vi "Dashboard Main.vi"() -> ()   [LabVIEW 2019]
uses:
  <vilib>/Utility/miscctls.llb/LVRowAndColumnTypeDef.ctl
  <vilib>/event_ctls.llb/eventvkey.ctl
  <vilib>/Rock Robotics/Network Tables/NT Read Numeric Array.vi
  <vilib>/Rock Robotics/WPI/Dashboard/WPI_DashboardLogging Global.vi
  <vilib>/Rock Robotics/Network Tables/NT Read Boolean.vi
  <vilib>/Rock Robotics/Network Tables/NT Write Boolean.vi
panel:
  in  "Camera Settings Right":T1={"Frame Rate"=30, "Compression"=30, "Size"=1, "DB Camera Config"=FALSE} {"Frame Rate" scale=1.0..30.0; "Compression" scale=100.0..-1.0; "Size" items=["640x480", "320x240", "160x120"]}
  in  "Camera Name Right":string(combo)="No Camera Selection"
  out "Camera Perf":string
  in  "Camera Settings":T1={"Frame Rate"=30, "Compression"=30, "Size"=1, "DB Camera Config"=FALSE} {"Frame Rate" scale=1.0..30.0; "Compression" scale=100.0..-1.0; "Size" items=["640x480", "320x240", "160x120"]}
  in  "TCP":refnum<k5>
  in  "Rec Mode":enum32{"Stop", "Record", "Playback"}(radio)
  out "Robot IP":string
  out "Image Message":string="Timeout in Camera Communications"
  in  "Dashboard Tab":T2(tab)
  in  "Dual Operators?":bool=TRUE
  in  "FT to IN":bool
  out "Target Acquired":bool
  out "Vision Enabled":bool
  out "NT Connection":bool
  out "MotorChart R":cluster{"Numeric":dbl, "Numeric":dbl}(graph)
  out "MotorChart L":cluster{"Numeric":dbl, "Numeric":dbl}(graph)
  out "MotorSliders R":cluster{"MotorSlide1":dbl, "MotorSlide2":dbl} {"MotorSlide2" scale=-1.0..1.0 scale format="%#_2e"; "MotorSlide1" scale=-1.0..1.0 scale format="%#_2e"}
  out "MotorSliders L":cluster{"MotorSlide1":dbl, "MotorSlide2":dbl} {"MotorSlide2" scale=-1.0..1.0 scale format="%#_2e"; "MotorSlide1" scale=-1.0..1.0 scale format="%#_2e"}
  out "JS1 Z":dbl(slide) scale=-1.0..1.0 scale format="%#_2e"
  out "JS1 Graph":cluster{"X":dbl, "Y":dbl}[](graph)
  out "JS1 Buttons":T3
  out "JS2 Z":dbl(slide) scale=-1.0..1.0 scale format="%#_2e"
  out "JS2 Graph":cluster{"X":dbl, "Y":dbl}[](graph)
  out "JS2 Buttons":T3
  out "Mode":T4(ring)=enum."Auto Disabled"
  out "Right Camera Perf":cluster{"Bandwidth (Mbps)":dbl, "FPS":dbl}
  in  "Select Auto":string(combo)="Select Autonomous ..."
  out "Target Distance":dbl
  out "Camera Image Right":T5(plugin-control)
  out "Skew":dbl caption="DB/String 1"
  out "Area":dbl caption="DB/String 1"
  out "Offset X":dbl
  out "Offset Y":dbl
  out "Bottom RPM":dbl caption="DB/String 1"
  out "Top RPM":dbl caption="DB/String 1"
  in  "Test Slider":dbl(slide) scale=0.0..100.0 scale format="%#_3g"
  in  "On/Off":bool caption="Solenoid"
  in  "Test Name":u16(ring) items=["Select the test to run..."]
  in  "Test Tree":string(tree)
  in  "Motor":cluster{"Value":dbl, "Enable":bool} {"Value" scale=-1.0..1.0 scale format="%#_3g"}
  out "Progress":T6 {"Test Progress" scale=0.0..100.0}
  in  "Rev/Fwd":cluster{"Forward":bool, "Reverse":bool}
  in  "Test Ring":u16(ring) items=["Monochrome", "Color"]
  out "Cmd Status":string
  in  "Execute Command":bool
  in  "Command Params":string[][](table)
  in  "Command Selection":i32(listbox)
  in  "CheckList":i32(listbox)
  out "Tree":string(tree)
  out "Camera Image":T5(plugin-control)
  out "Background":bool
  in  "Camera Name":string(combo)="No Camera Selection"
  # "HW"
  # "HW"
  # "Drive Motors"
  # "Front"
  # "Operator 1"
  # "Operator 2"
  # "Right"
  # "Left"
  # "Back"
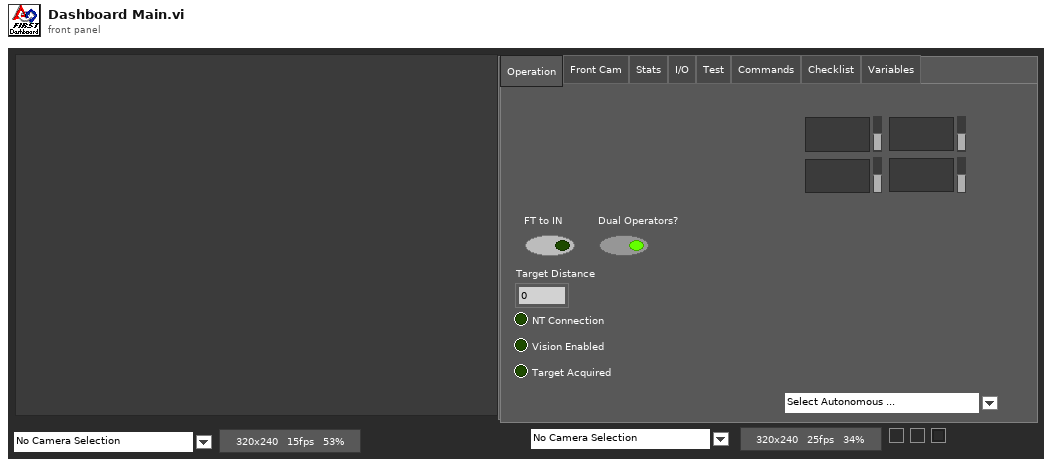
[diagram p1: front panel]
types:
  T1 = cluster{"Frame Rate":i32, "Compression":i32, "Size":u16, "DB Camera Config":bool}
  T2 = enum32{"Operation", "Front Cam", "Stats", "I/O", "Test", "Commands", "Checklist", "Variables"}
  T3 = cluster{bool, bool, bool, bool, bool, bool, bool, bool, bool, bool, bool, bool}
  T4 = enum8{"Tele-Op Disabled", "Tele-Op Enabled", "Auto Disabled", "Auto Enabled", "Test Disabled", "Test Enabled", "Disconnected", "No Code", "E-Stop"}
  T5 = typedef "IMAQ Image.ctl" = refnum<image>
  T6 = cluster{"Test Progress":u8, "Test Progress Text":string}
  T7 = cluster{"Save Path":path, "Interval (s)":dbl, "Keep":i32}
  T8 = enum32{"Drive", "Camera", "Basic", "Custom", "Test", "Commands", "Checklist", "Variables"}
  T9 = typedef "Image Type" = u32
  T10 = cluster{"IDs":cluster{"RPC field ID":u16, "Unique ID":u16}, "String":string}
  T11 = cluster{"Camera Image":refnum<vi>, "Dashboard Tab":refnum<vi>, "Background":refnum<vi>, "Rec Mode":refnum<vi>, "Test Slider":refnum<vi>, "On/Off ":refnum<vi>, "Test Ring":refnum<vi>, "Rev/Fwd":refnum<vi>, "Test Name":refnum<vi>, "Motor":refnum<vi>, "Progress":refnum<vi>, "CheckList":refnum<vi>, "Tree":refnum<vi>, "Test Tree":refnum<vi>, "Command Params":refnum<vi>, "Command Selection":refnum<vi>, "Execute Command":refnum<vi>, "Cmd Status":refnum<vi>, "Camera Settings":refnum<vi>, "Camera Name":refnum<vi>, "Camera Perf":refnum<vi>, "Camera Settings Right":refnum<vi>, "Camera Name Right":refnum<vi>, "Camera Image Right":refnum<vi>}
  T12 = cluster{"Global Rectangle":i32[], "Contours":cluster{"Contour Type":u32, "ROI Type":u32, "Points":i32[]}[]}
  T13 = cluster{"Camera Name Right":string, string, "Saved DB Images Info":cluster{"Save Path":path, "Interval (s)":dbl, "Keep":i32}}
  T14 = cluster{"Error Strings":string, "Disable Counts":cluster{u16, u16}, "Rail Faults":cluster{u16, u16, u16}, "Robot IP":string, "DB Mode":u8, "Event Info":cluster{"Name":string, "Type":u8, "Number":u16, "Replay":u8}}
  T15 = cluster{"Storage":cluster{"Disk Free":u64, "RAM Block":u32, "RAM free":u32}, "CPU Utilization":cluster{"CPU % ISR":sgl, "CPU % Time Crit":sgl, "CPU % Timed Str":sgl, "CPU % High":sgl, "CPU % Above":sgl, "CPU % Normal":sgl, "CPU % Low":sgl}, "CAN":cluster{"% Bus Utilization":sgl, "Bus Off Cnt":u32, "TX_FIFO Full Cnt":u32, "Receive Error Cnt":u8, "Transmit Error Cnt":u8}, "HID":cluster{"HID Outputs":u32, "Rumble Low":u16, "Rumble High":u16}[]}
  T16 = cluster{"Status bits":cluster{"Test Mode":bool, "Autonomous":bool, "Enabled":bool, "Code Start":bool, "Brownout":bool, "Reserved 2":bool, "Reserved 3":bool, "E-Stop":bool}, "Code Trace":cluster{"Disabled":bool, "TeleOp":bool, "Auto":bool, "Test":bool}, "Controller Type":enum16{"unknown", "cRIO", "roboRio"}, "Code?":enum16{"unknown", "noCode", "code"}, "Battery V":dbl}
  T17 = cluster{"Control Bits":cluster{"TestMode":bool, "Autonomous":bool, "Enabled":bool, "FMS Present":bool, bool, bool, bool, "E-Stop":bool}, "Team Station ":u8, "Countdown":sgl, "Joystick Values":cluster{"Axes":dbl[], "Buttons":bool[], "POVs":i16[]}[]}
  T18 = cluster{"Axes":dbl[], "Buttons":bool[], "POVs":i16[]}[]
  T19 = cluster{"Axes":dbl[], "Buttons":bool[], "POVs":i16[]}
  T20 = cluster{"Buttons[0]":bool, "Buttons[1]":bool, "Buttons[2]":bool, "Buttons[3]":bool, "Buttons[4]":bool, "Buttons[5]":bool, "Buttons[6]":bool, "Buttons[7]":bool, "Buttons[8]":bool, "Buttons[9]":bool, "Buttons[10]":bool, "Buttons[11]":bool}
  T21 = cluster{"Camera Name":string, string, "Saved DB Images Info":cluster{"Save Path":path, "Interval (s)":dbl, "Keep":i32}}
  T22 = cluster{"Operation":enum16{"Update", "Clear"}, "Color Box":u32}[]
  T23 = typedef "eventvkey.ctl" = enum16{"ASCII", "Enter", "Return", "Shift", "Ctrl", "Alt", "Cmd", "Opt", "Caps", "NumLock", "Clear", "Break", "Up", "Down", "Left", "Right", "Insert", "Delete", "Home", "End", "PageUp", "PageDown", "Escape", "Help", "Pause", "ScrollLock", "F1", "F2", "F3", "F4", "F5", "F6", "F7", "F8", "F9", "F10", "F11", "F12", "F13", "F14", "F15", "F16", "F17", "F18", "F19", "F20", "F21", "F22", "F23", "F24", "Play", "VolumeUp", "VolumeDown", "Mute", "Two Byte Char"}
  T24 = cluster{"Image Size":bool, "Image Type":bool, "Pixel Value":bool, "ROI Information":bool, "Zoom Factor":bool}
  T25 = cluster{"Operation":enum16{"Update", "Clear"}, "Color Box":u32}
  T26 = typedef "LVRowAndColumnTypeDef.ctl" = cluster{"Row":i32, "Column":i32}
  T27 = cluster{"Shift":bool, "Ctrl":bool, "Alt":bool, "Cmd":bool, "Opt":bool}
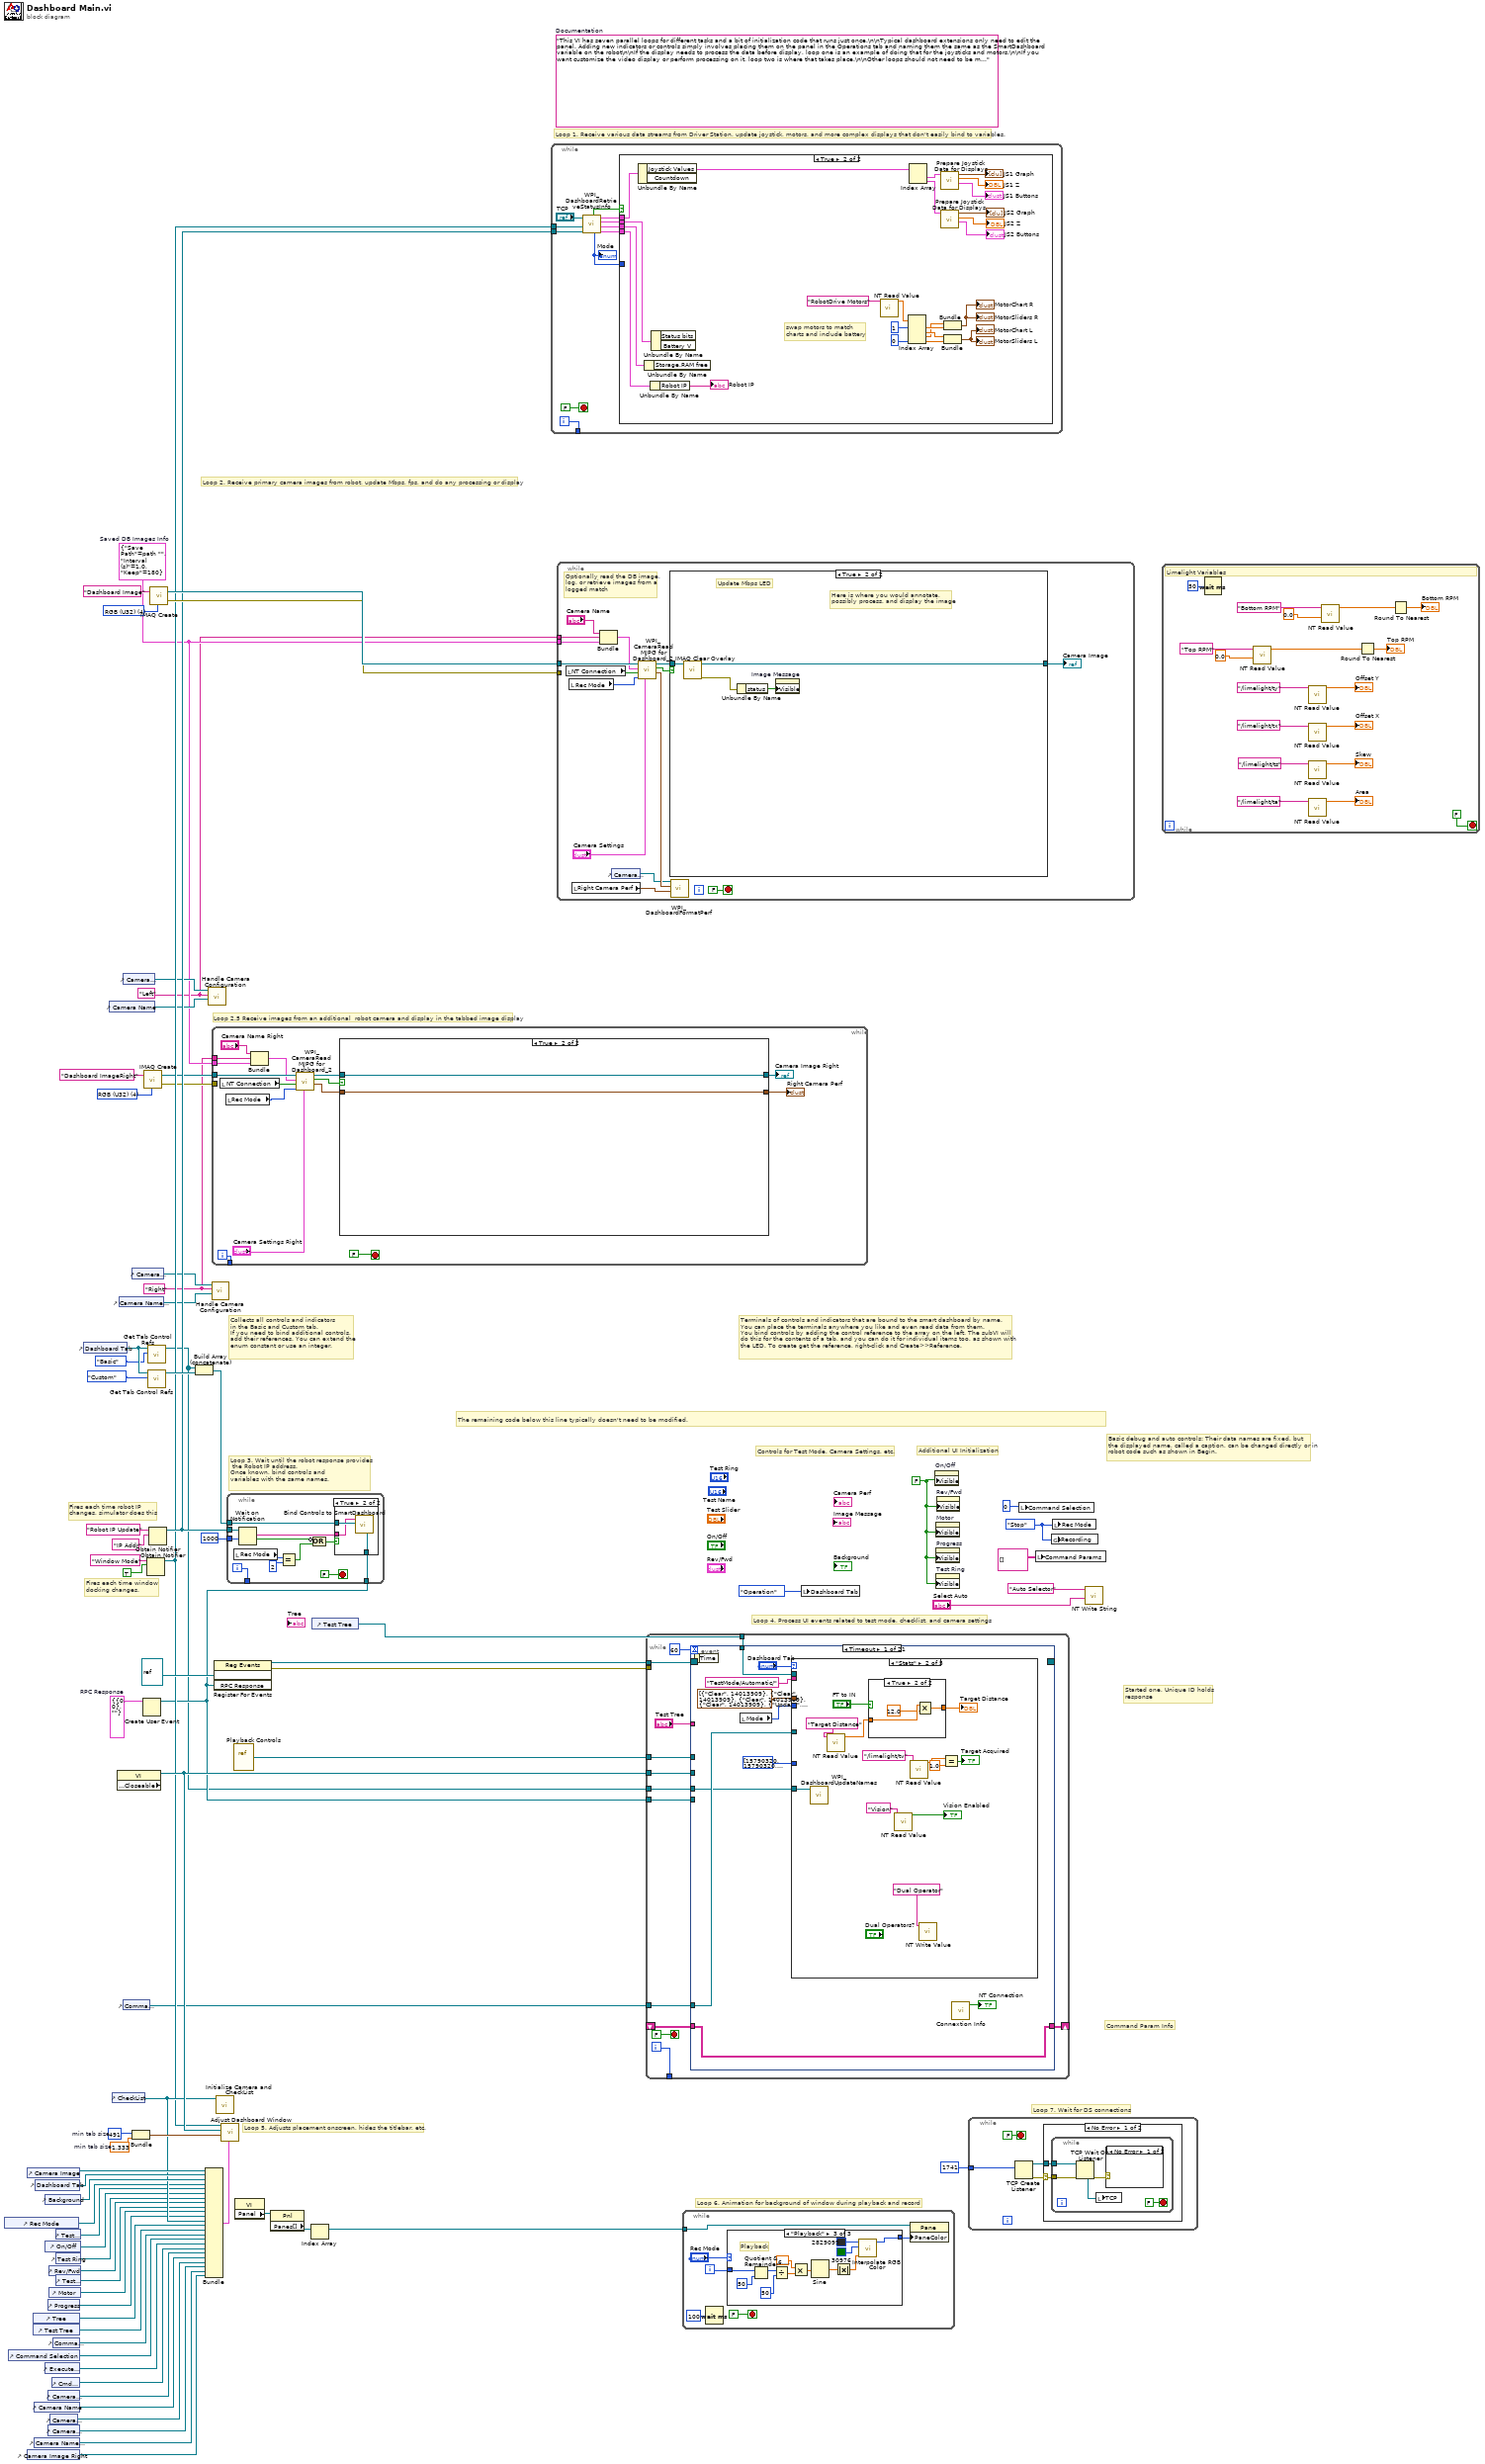
[diagram p0: block diagram]
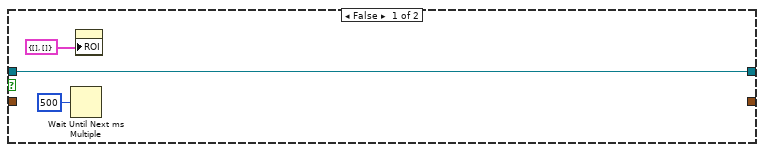
[diagram p2: hidden frame]
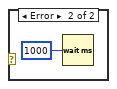
[diagram p3: hidden frame]
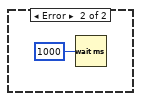
[diagram p4: hidden frame]
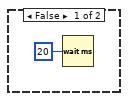
[diagram p5: hidden frame]
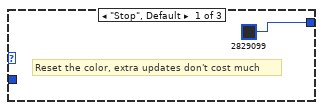
[diagram p6: hidden frame]
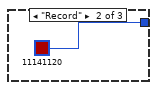
[diagram p7: hidden frame]
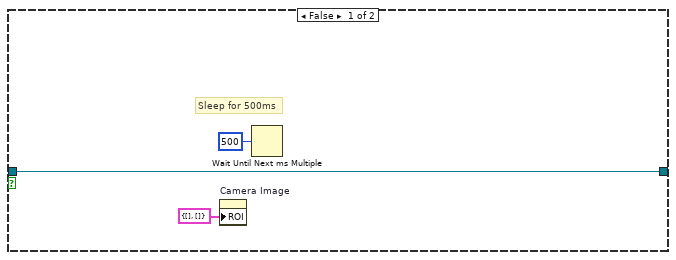
[diagram p9: hidden frame]
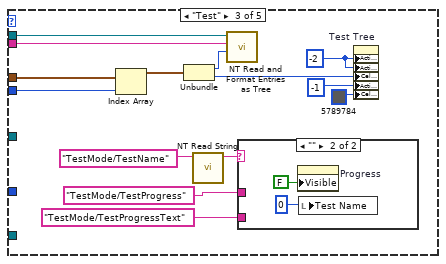
[diagram p12: hidden frame]
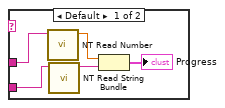
[diagram p13: hidden frame]
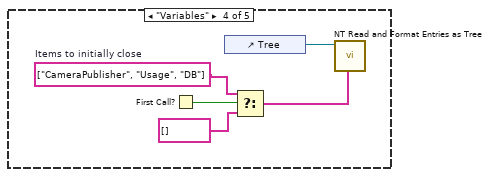
[diagram p14: hidden frame]
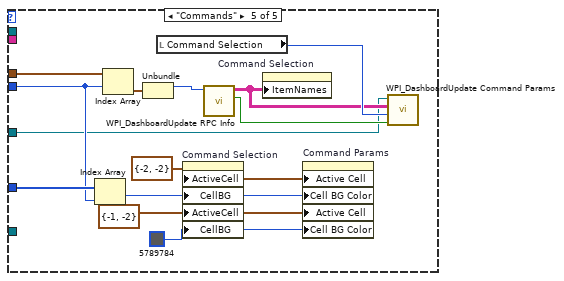
[diagram p15: hidden frame]
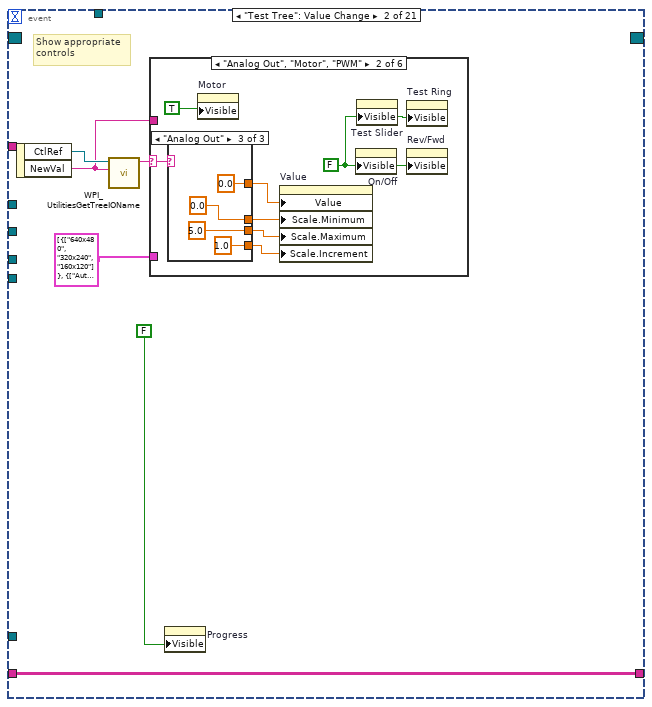
[diagram p16: hidden frame]
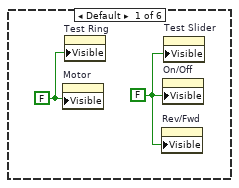
[diagram p17: hidden frame]
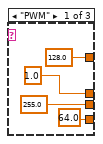
[diagram p18: hidden frame]
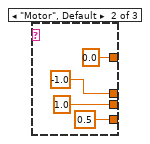
[diagram p19: hidden frame]
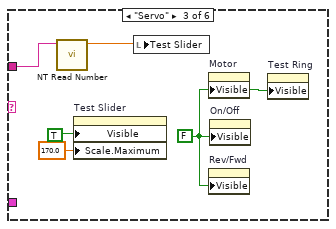
[diagram p20: hidden frame]
diagram:
  w4 = T7 {"Save Path"=path "", "Interval (s)"=1.0, "Keep"=180}  # Saved DB Images Info
  w3 = "Right"
  w2 = "Left"
  w14 = T9 4 items=["Grayscale (U8)", "Grayscale (I16)", "Grayscale (SGL)", "Complex (CSG)", "RGB (U32)", "HSL (U32)", "RGB (U64)"] ("Image Type")
  w30 = T10 {"IDs"={"RPC field ID"=0, "Unique ID"=0}, "String"=""}  # RPC Response
  w52 = 491  # min tab size
  w51 = 1.333  # min tab size
  w59 = enum32{"Stop", "Record", "Playback"}."Stop" ("Rec Mode")
  w36 = FALSE ("Visible")
  (unwired) "This VI has seven parallel loops for different tasks and a bit of initialization code that runs just once.\n\nTypical dashboard extensions only need to edit the panel. Adding new indicators or controls simply involves placing them on the panel in the Operations tab and naming them the same as the SmartDashboard variable on the robot\n\nIf the display needs to process the data before display, loop one is an example of doing that for the joysticks and motors.\n\nIf you want customize the video display or perform processing on it, loop two is where that takes place.\n\nOther loops should not need to be modified. They are pretty standard, and document the task they perform."  # Documentation
  w76 = T9 4 items=["Grayscale (U8)", "Grayscale (I16)", "Grayscale (SGL)", "Complex (CSG)", "RGB (U32)", "HSL (U32)", "RGB (U64)"] ("Image Type")
  # "Loop 2.5 Receive images from an additional  robot camera and display in the tabbed image display"
  # "Command Param Info"
  # "Started one, Unique ID holds\nresponse"
  # "Loop 7. Wait for DS connections"
  # "Basic debug and auto controls: Their data names are fixed, but\nthe displayed name, called a caption, can be changed directly or in\nrobot code such as shown in Begin."
  # "Controls for Test Mode, Camera Settings, etc."
  # "Additional UI Initialization"
  # "Loop 6. Animation for background of window during playback and record"
  # "Fires each time robot IP\nchanges, simulator does this"
  # "Fires each time window\ndocking changes."
  # "Collects all controls and indicators\nin the Basic and Custom tab.\nIf you need to bind additional controls,\nadd their references. You can extend the\nenum constant or use an integer."
  # "The remaining code below this line typically doesn't need to be modified."
  # "Loop 4. Process UI events related to test mode, checklist, and camera settings"
  # "Terminals of controls and indicators that are bound to the smart dashboard by name.\nYou can place the terminals anywhere you like and even read data from them.\nYou bind controls by adding the control reference to the array on the left. The subVI will\ndo this for the contents of a tab, and you can do it for individual items too, as shown with\nthe LED. To create get the reference, right-click and Create>>Reference."
  # "Loop 3. Wait until the robot response provides\n the Robot IP address.\nOnce known, bind controls and\nvariables with the same names."
  # "Loop 5. Adjusts placement onscreen, hides the titlebar, etc."
  # "Loop 1. Receive various data streams from Driver Station, update joystick, motors, and more complex displays that don't easily bind to variables."
  # "Loop 2. Receive primary camera images from robot, update Mbps, fps, and do any processing or display"
  n1 = control-ref of="Rec Mode"() -> (w42:refnum<vi>)
  n2 = control-ref of="Command Selection"() -> (w29:refnum<vi>)
  n3 = control-ref of="Camera Image Right"() -> (w7:refnum<vi>)
  n4 = control-ref of="Camera Image"() -> (w54:refnum<vi>)
  n5 = control-ref of="Tree"() -> (w46:refnum<vi>)
  n6 = control-ref of="Test Tree"() -> (w45:refnum<vi>)
  n7 = control-ref of="Camera Name"() -> (w20:refnum<vi>)
  n8 = control-ref of="Camera Name Right"() -> (w8:refnum<vi>)
  n9 = control-ref of="Dashboard Tab"() -> (w53:refnum<vi>)
  n10 = control-ref of="Execute Command"() -> (w31:refnum<vi>)
  n11 = control-ref of="Background"() -> (w49:refnum<vi>)
  n12 = control-ref of="On/Off"() -> (w40:refnum<vi>)
  n13 = control-ref of="Progress"() -> (w37:refnum<vi>)
  n14 = control-ref of="Camera Settings"() -> (w21:refnum<vi>)
  n15 = control-ref of="Camera Settings Right"() -> (w9:refnum<vi>)
  n16 = control-ref of="Rev/Fwd"() -> (w38:refnum<vi>)
  n17 = control-ref of="Motor"() -> (w43:refnum<vi>)
  n18 = control-ref of="Camera Perf"() -> (w19:refnum<vi>)
  n19 = control-ref of="Cmd Status"() -> (w25:refnum<vi>)
  n20 = control-ref of="Command Params"() -> (w32:refnum<vi>)
  n21 = control-ref of="Test Slider"() -> (w41:refnum<vi>)
  n22 = control-ref of="Test Ring"() -> (w39:refnum<vi>)
  n23 = control-ref of="Test Name"() -> (w44:refnum<vi>)
  n24 = control-ref of="Dashboard Tab"() -> (w57:refnum<vi>)
  n25 = control-ref of="Camera Name"() -> (w22:refnum<vi>)
  n26 = control-ref of="CheckList"() -> (w47:refnum<vi>)
  n27 = property class="VI" props=["Front Panel.Closeable"]() -> (reference out=w58:refnum<vi>)  [unwired: 2 in, 2 out]
  n28 = control-ref of="Camera Name Right"() -> (w10:refnum<vi>)
  n29 = control-ref of="Camera Settings"() -> (w23:refnum<vi>)
  n30 = control-ref of="Command Params"() -> (w24:refnum<vi>)
  n31 = control-ref of="Camera Settings Right"() -> (w11:refnum<vi>)
  n32 = Bundle("min tab size"=w52, "min tab size"=w51) -> (w50:cluster{"min tab size":i32, "min tab size":dbl})  [unwired: 1 in]
  n33 = Create User Event(user event datatype=w30) -> (user event=w26:refnum<user-event>)  [unwired: 1 in, 1 out]
  n34 = call "IMAQ Create"("Image Name"="Dashboard ImageRight", "Image Type"=w14) -> ("New Image"=w13:T5, "error out"=w12:errorcluster)  [unwired: 2 in, 1 out]
  n35 = Obtain Notifier(name (unnamed)="Window Mode", notification data type=TRUE) -> (notifier out=w34:refnum<notifier>)  [unwired: 2 in, 2 out]
  n36 = call <vilib>:"Get Tab Control Refs.vi"("Page Index"=T8."Basic" ("Dashboard Tab"), "TabControl in"=w57) -> ("ControlsOnPage"=w18:refnum<vi>[])  [unwired: 9 in]
  n37 = call <vilib>:"Get Tab Control Refs.vi"("Page Index"=T8."Custom" ("Dashboard Tab"), "TabControl in"=w57) -> ("ControlsOnPage"=w56:refnum<vi>[])  [unwired: 9 in]
  n38 = Obtain Notifier(name (unnamed)="Robot IP Update", notification data type="IP Addr" ("name (unnamed)")) -> (notifier out=w35:refnum<notifier>)  [unwired: 2 in, 2 out]
  n39 = call "IMAQ Create"("Image Name"="Dashboard Image", "Image Type"=w76) -> ("New Image"=w74:T5, "error out"=w73:errorcluster)  [unwired: 2 in, 1 out]
  n40 = Build Array (concatenate)(w18, w56) -> (w55:refnum<vi>[])
  n41 = Bundle("Camera Image"=w54, "Dashboard Tab"=w53, "Background"=w49, "Rec Mode"=w42, "Test Slider"=w41, "On/Off"=w40, "Test Ring"=w39, "Rev/Fwd"=w38, "Test Name"=w44, "Motor"=w43, "Progress"=w37, "CheckList"=w47, "Tree"=w46, "Test Tree"=w45, "Command Params"=w32, "Command Selection"=w29, "Execute Command"=w31, "Cmd Status"=w25, "Camera Settings"=w21, "Camera Name"=w20, "Camera Perf"=w19, "Camera Settings Right"=w9, "Camera Name Right"=w8, "Camera Image Right"=w7) -> (w48:T11)  [unwired: 1 in]
  n42 = call "Handle Camera Configuration.vi"("CameraNameRef"=w22, "Display Name"=w2, "ClusterRef"=w23) -> ()  [unwired: 9 in]
  n43 = call "Handle Camera Configuration.vi"("CameraNameRef"=w10, "Display Name"=w3, "ClusterRef"=w11) -> ()  [unwired: 9 in]
  n44 = while {
    tunnel: w13 -> [w91]
    tunnel: w12 -> [_]
    tunnel: [w86] -> _
    tunnel: w4 -> [w83]
    tunnel: w3 -> [w80]
    i -> [w86]
    stop <- FALSE stop-if-true
    n45 = local read "NT Connection"() -> (w84:bool)
    n46 = local read "Rec Mode"() -> (w90:enum32{"Stop", "Record", "Playback"})
    n47 = Bundle("Camera Name Right"="Camera Name Right", w80, "Saved DB Images Info"=w83) -> (w82:T13)  [unwired: 1 in]
    n48 = call <vilib>:"WPI_CameraRead MJPG for Dashboard_2.vi"("Camera Settings"="Camera Settings Right", "Rec Mode"=w90, "NT Connection"=w84, "Capture Info"=w82, "Image in"=w91) -> ("perf info"=w78:cluster{"Bandwidth (Mbps)":dbl, "fps":dbl}, "Active"=w85:bool, "Image\\ out"=w88:T5)  [unwired: 4 in]
    n49 = case shown="True" w85 {
      tunnel: w88 -> [w93 w95]
      tunnel: [w93 w95] -> w77
      tunnel: [_ w96] -> w79
      tunnel: w78 -> [_ w96]
      frame False {
        n50 = Wait Until Next ms Multiple(millisecond multiple=u32 500) -> ()  [unwired: 1 out]
        n51 = property on="Camera Image Right" class="ImageControl"("ROI"=T12 {"Global Rectangle"=[], "Contours"=[]}) -> ()  [unwired: 2 in, 2 out]
      }
      frame True {
      }
    }
    "Right Camera Perf" <- w79
    "Camera Image Right" <- w77
  }
  n52 = register-events(refnum<vi> refnum, w26) -> (reference out=w63:refnum<event-registration>, error out=w62:errorcluster)  [unwired: 2 in]
  n53 = call "Initialize Camera and CheckList.vi"("ListBox in"=w47) -> ()  [unwired: 11 in]
  n54 = call "Adjust Dashboard Window.vi"("Sizing Refnums"=w48, "Size Constraints"=w50, "VI"=w58, "WIn Mode"=w34) -> ()  [unwired: 8 in]
  n55 = while {
    tunnel: w55 -> [w108]
    tunnel: w35 -> [w106]
    tunnel: [w104] -> _
    tunnel: u32 1000 ("milliseconds to wait") -> [w103]
    tunnel: w26 -> [w97]
    i -> [w104]
    stop <- FALSE stop-if-true
    n56 = local read "Rec Mode"() -> (w99:enum32{"Stop", "Record", "Playback"})
    n57 = Wait on Notification(notifier=w106, timeout in ms (-1)=w103) -> (notification=w105:string, timed out?=w101:bool)  [unwired: 2 in, 2 out]
    n58 = Equal?(x=w99, y=u16 2 ("Rec Mode")) -> (x = y?=w100:bool)
    n59 = Compound Arithmetic op=OR(invert w101, w100) -> (w102:bool)
    n60 = case shown="True" w102 {
      tunnel: w108 -> [_ w111]
      tunnel: w105 -> [_ w110]
      tunnel: w97 -> [_ w109]
      frame False {
      }
      frame True {
        n61 = call <vilib>:"Bind Controls to SmartDashboard.vi"("RPC ref"=w109, "Bound Control Refs"=w111, "Server IP Address"=w110) -> ()  [unwired: 9 in]
      }
    }
  }
  n62 = vi-ref "Playback Controls.vi"() -> (w64:refnum<vi>)
  n63 = property class="VI"() -> ("Panel"=w66:refnum<vi>)  [unwired: 2 in, 2 out]
  n64 = property class="Pnl"(reference=w66) -> ("Panes[]"=w67:refnum<vi>[])  [unwired: 1 in, 2 out]
  n65 = Index Array(array=w67) -> (element=w65:refnum<vi>)  [unwired: 1 in]
  n66 = control-ref of="Test Tree"() -> (w68:refnum<vi>)
  n67 = while {
    tunnel: [w121] -> _
    tunnel: w35 -> [w115]
    tunnel: w34 -> [w112]
    i -> [w121]
    stop <- FALSE stop-if-true
    n68 = call <vilib>:"WPI_DashboardRetrieveStatusInfo.vi"("Binding Refnum"=w115, "Window Mode Notifier"=w112, "TCP Cnx"="TCP") -> ("Power and Errors"=w116:T14, "Robot Metrics"=w119:T15, "Status Info"=w120:T16, "Control Info"=w117:T17, "Robot Mode"=w114:T4, "Process?"=w118:bool)  [unwired: 3 in]
    "Mode" <- w114
    n69 = case shown="True" w118 {
      tunnel: w120 -> [_ w147]
      tunnel: w119 -> [_ w146]
      tunnel: w117 -> [_ w145]
      tunnel: w116 -> [_ w144]
      tunnel: w114 -> [_ _]
      frame False {
        n70 = Wait (ms)(milliseconds to wait=u32 20) -> ()  [unwired: 1 out]
      }
      frame True {
        # "swap motors to match\ncharts and include battery"
        n71 = Unbundle By Name(w145) -> ("Joystick Values"=w135:T18)  [unwired: 1 out]
        n72 = Unbundle By Name(w146) -> ()  [unwired: 1 out]
        n73 = Unbundle By Name(w144) -> ("Robot IP"=→"Robot IP":string)
        n74 = Unbundle By Name(w147) -> ()  [unwired: 2 out]
        n75 = call-poly <vilib>:"NT Read Value.vi"("Name"="RobotDrive Motors") -> ("Numeric Array"=w125:dbl[])  [unwired: 9 in, 1 out]
        n76 = Index Array(array=w125, index #1=1, index #4=0) -> (element #1=w139:dbl, element #2=w140:dbl, element #3=w138:dbl, element #4=w143:dbl)  [unwired: 2 in]
        n77 = Index Array(array=w135) -> (element #1=w134:T19, element #2=w130:T19)  [unwired: 2 in]
        n78 = call "Prepare Joystick Data for Displays.vi"("Joystick Values"=w130) -> ("Buttons"=→"JS2 Buttons":T20, "Z Axis"=→"JS2 Z":dbl, "Cartesian Data"=→"JS2 Graph":cluster{"X axis":dbl, "X axis":dbl}[])  [unwired: 8 in]
        n79 = call "Prepare Joystick Data for Displays.vi"("Joystick Values"=w134) -> ("Buttons"=→"JS1 Buttons":T20, "Z Axis"=→"JS1 Z":dbl, "Cartesian Data"=→"JS1 Graph":cluster{"X axis":dbl, "X axis":dbl}[])  [unwired: 8 in]
        n80 = Bundle("Numeric"=w138, "Numeric"=w139) -> (→"MotorChart R" →"MotorSliders R":cluster{"Numeric":dbl, "Numeric":dbl})  [unwired: 1 in]
        n81 = Bundle("Numeric"=w140, "Numeric"=w143) -> (→"MotorChart L" →"MotorSliders L":cluster{"Numeric":dbl, "Numeric":dbl})  [unwired: 1 in]
      }
    }
  }
  n82 = while {
    tunnel: w74 -> [w161]
    tunnel: w73 -> [_]
    tunnel: w4 -> [w155]
    tunnel: w2 -> [w152]
    stop <- FALSE stop-if-true
    # "Optionally read the DB image,\nlog, or retrieve images from a\nlogged match"
    n83 = local read "NT Connection"() -> (w156:bool)
    n84 = local read "Rec Mode"() -> (w158:enum32{"Stop", "Record", "Playback"})
    n85 = local read "Right Camera Perf"() -> (w150:cluster{"Bandwidth (Mbps)":dbl, "FPS":dbl})
    n86 = Bundle("Camera Name"="Camera Name", w152, "Saved DB Images Info"=w155) -> (w154:T21)  [unwired: 1 in]
    n87 = control-ref of="Camera Perf"() -> (w149:refnum<vi>)
    n88 = call <vilib>:"WPI_CameraRead MJPG for Dashboard_2.vi"("Camera Settings"="Camera Settings", "Rec Mode"=w158, "NT Connection"=w156, "Capture Info"=w154, "Image in"=w161) -> ("perf info"=w151:cluster{"Bandwidth (Mbps)":dbl, "fps":dbl}, "Active"=w159:bool, "Image\\ out"=w160:T5)  [unwired: 4 in]
    n89 = case shown="True" w159 {
      tunnel: w160 -> [w164 w167]
      tunnel: [w164 w166] -> w148
      frame False {
        # "Sleep for 500ms"
        n90 = property on="Camera Image" class="ImageControl"("ROI"=T12 {"Global Rectangle"=[], "Contours"=[]}) -> ()  [unwired: 2 in, 2 out]
        n91 = Wait Until Next ms Multiple(millisecond multiple=u32 500) -> ()  [unwired: 1 out]
      }
      frame True {
        # "Here is where you would annotate,\npossibly process, and display the image"
        # "Update Mbps LED"
        n92 = call "IMAQ Clear Overlay"("Image"=w167) -> ("error out"=w168:errorcluster, "Image Out"=w166:T5)  [unwired: 2 in, 7 out]
        n93 = Unbundle By Name(w168) -> ("status"=w169:bool)
        n94 = property on="Image Message" class="Str"("Visible"=w169) -> ()  [unwired: 2 in, 2 out]
      }
    }
    "Camera Image" <- w148
    n95 = call <vilib>:"WPI_DashboardFormatPerf.vi"("Right Camera Perf"=w150, "Performance"=w151, "String in"=w149) -> ()  [unwired: 9 in]
  }
  n96 = while {
    tunnel: [w179] -> _
    tunnel: w68 -> [w178]
    tunnel: w64 -> [w177]
    tunnel: w63 -> [w176]
    tunnel: w62 -> [_]
    tunnel: w58 -> [w175]
    tunnel: w26 -> [w174]
    tunnel: w24 -> [w173]
    shift-right: [w172] -> _
    shift-left: _ -> [w171]
    tunnel: w18 -> [w170]
    i -> [w179]
    stop <- FALSE stop-if-true
    n97 = event shown="[0] Timeout" {
      selector: w176 -> [_ _ _ _ _ _ _ _ _ _ _ _ _ _ _ _ _ _ _ _ _]
      dyn-events: [_ _ _ _ _ _ _ _ _ _ _ _ _ _ _ _ w454 _ _ _ _] -> _
      timeout: u32 60 ("milliseconds to wait") -> [_ _ _ _ _ _ _ _ _ _ _ _ _ _ _ _ _ _ _ _ _]
      tunnel: w178 -> [w191 _ _ _ _ _ _ _ _ _ _ _ _ _ _ _ _ _ _ _ _]
      tunnel: "Test Tree" -> [_ _ _ _ _ _ _ _ _ _ _ w421 w429 w431 w435 w443 _ _ _ _ _]
      tunnel: w177 -> [_ _ _ _ _ _ _ _ _ _ _ _ _ _ _ _ w456 _ w474 _ _]
      tunnel: w175 -> [_ _ _ _ _ _ _ _ _ _ _ _ _ _ _ _ w452 _ _ _ _]
      tunnel: w174 -> [_ _ _ _ _ _ _ _ _ _ _ _ _ _ _ _ w450 _ _ _ _]
      tunnel: w173 -> [w186 _ _ _ _ _ w372 _ _ _ _ _ _ _ _ _ _ _ _ _ _]
      tunnel: [w185 w249 w351 w356 w365 w369 w370 w379 w389 w396 w408 w420 w427 w430 w434 w442 w449 w469 w471 w475 w488] -> w172
      tunnel: w171 -> [w185 w249 w351 w356 w365 w369 w370 _ _ w396 w408 w420 w427 w430 w434 w442 w449 w469 w471 w475 w488]
      tunnel: w170 -> [w183 _ _ _ _ _ _ _ _ _ _ _ _ _ _ _ _ _ _ _ _]
      event Timeout {
        n98 = event-data() -> ()  [unwired: 1 in, 1 out]
        n99 = local read "Mode"() -> (w188:T4)
        n100 = case shown="\"Stats\"" "Dashboard Tab" {
          tunnel: w191 -> [_ _ w222 _ _]
          tunnel: "TestMode/Automatic/" ("Name Pattern") -> [_ _ w221 _ _]
          tunnel: T22 [{"Operation"=enum."Clear", "Color Box"=14013909}, {"Operation"=enum."Clear", "Color Box"=14013909}, {"Operation"=enum."Clear", "Color Box"=14013909}, {"Operation"=enum."Clear", "Color Box"=14013909}, {"Operation"=enum."Update", "Color Box"=14013909}, {"Operation"=enum."Update", "Color Box"=16777215}, {"Operation"=enum."Clear", "Color Box"=14013909}, {"Operation"=enum."Clear", "Color Box"=14013909}, {"Operation"=enum."Clear", "Color Box"=14013909}] -> [_ _ w214 _ w242]
          tunnel: w188 -> [_ _ w213 _ w241]
          tunnel: u32[] [15790320, 15790320, 15790320, 15790320, 16777215, 16777215, 15790320, 15790320, 15790320] -> [_ _ _ _ w247]
          tunnel: w186 -> [_ _ _ _ w235]
          tunnel: w183 -> [_ w204 _ _ _]
          frame "I/O", Default {
          }
          frame "Stats" {
            n101 = call <vilib>:"WPI_DashboardUpdateNames.vi"("Controls on Tab"=w204) -> ()  [unwired: 11 in]
            n102 = call-poly <vilib>:"NT Read Value.vi"("Name"="Target Distance") -> ("Numeric"=w202:dbl)  [unwired: 9 in, 1 out]
            n103 = case shown="True" "FT to IN" {
              tunnel: w202 -> [w205 w207]
              tunnel: [w205 w208] -> w203
              frame False {
              }
              frame True {
                n104 = Multiply(x=w207, y=12.0) -> (x*y=w208:dbl)
              }
            }
            "Target Distance" <- w203
            n105 = call-poly <vilib>:"NT Read Value.vi"("Name"="Vision") -> ("Boolean"=→"Vision Enabled":bool)  [unwired: 9 in, 1 out]
            n106 = call-poly <vilib>:"NT Read Value.vi"("Name"="/limelight/tv") -> ("Numeric"=w198:dbl)  [unwired: 9 in, 1 out]
            n107 = call-poly <vilib>:"NT Write Value.vi"("Name"="Dual Operator") -> ()  [unwired: 10 in, 1 out]
            n108 = Equal?(x=w198, y=1.0) -> (x = y?=→"Target Acquired":bool)
          }
          frame "Test" {
            w220 = -2 ("Active Item:Row Number")
            n109 = Index Array(array=w214, index=w213) -> (element=w215:T25)
            n110 = Unbundle(w215) -> ("Operation"=w216:enum16{"Update", "Clear"}, "Color Box"=w217:u32)
            n111 = call <vilib>:"NT Read String.vi"("Name"="TestMode/TestName") -> ("String"=w211:string)  [unwired: 9 in, 1 out]
            n112 = call <vilib>:"NT Read and Format Entries as Tree.vi"("Operation"=w216, "Name Pattern"=w221, "Tree Refnum"=w222) -> ()  [unwired: 7 in, 2 out]
            n113 = case shown="\"\"" w211 {
              tunnel: "TestMode/TestProgress" ("Name") -> [w224 _]
              tunnel: "TestMode/TestProgressText" ("Name") -> [w223 _]
              frame Default {
                n114 = call <vilib>:"NT Read Number.vi"("Name"=w224) -> ("Numeric"=w225:dbl)  [unwired: 9 in, 1 out]
                n115 = call <vilib>:"NT Read String.vi"("Name"=w223) -> ("String"=w226:string)  [unwired: 9 in, 1 out]
                n116 = Bundle("Numeric"=w225, "String"=w226) -> (→"Progress":cluster{"Numeric":dbl, "String":string})  [unwired: 1 in]
              }
              frame "" {
                n117 = property on="Progress" class="Clust (strict)"("Visible"=FALSE) -> ()  [unwired: 2 in, 2 out]
                n118 = local write "Test Name"(u16 0) -> ()
              }
            }
            n119 = property on="Test Tree" class="Tree (strict)"("Active Item Row Number"=w220, "ActiveColNum"=w220, "CellBG"=w217, "Active Item Row Number"=-1 ("Active Item:Row Number"), "CellBG"=u32 5789784 ("Color Box")) -> ()  [unwired: 2 in, 2 out]
          }
          frame "Variables" {
            w232 = string[] ["CameraPublisher", "Usage", "DB"]  # Items to initially close
            n120 = First Call?() -> (First Call?: T/F=w233:bool)
            n121 = control-ref of="Tree"() -> (w234:refnum<vi>)
            n122 = Select(t=w232, s=w233, f=string[] []) -> (s? t:f=w230:string[])
            n123 = call <vilib>:"NT Read and Format Entries as Tree.vi"("Tags to  Close"=w230, "Tree Refnum"=w234) -> ()  [unwired: 8 in, 2 out]
          }
          frame "Commands" {
            w243 = u32 5789784 ("Color Box")
            w244 = T26 {"Row"=-1, "Column"=-2} ("Active Cell:Active Cell")
            w246 = T26 {"Row"=-2, "Column"=-2} ("Active Cell:Active Cell")
            n124 = Index Array(array=w247, index=w241) -> (element=w245:u32)
            n125 = Index Array(array=w242, index=w241) -> (element=w240:T25)
            n126 = Unbundle(w240) -> ("Operation"=w239:enum16{"Update", "Clear"})  [unwired: 1 out]
            n127 = local read "Command Selection"() -> (w238:i32)
            n128 = property on="Command Selection" class="MCListbox (strict)"("ActiveCell"=w246, "CellBG"=w245, "ActiveCell"=w244, "CellBG"=w243) -> ()  [unwired: 2 in, 2 out]
            n129 = call <vilib>:"WPI_DashboardUpdate RPC Info.vi"("Operation"=w239) -> ("update"=w237:bool, "commands"=w236:string[][])  [unwired: 9 in]
            n130 = property on="Command Selection" class="MCListbox (strict)"("ItemNames"=w236) -> ()  [unwired: 2 in, 2 out]
            n131 = property on="Command Params" class="Tbl (strict)"("Active Cell"=w246, "Cell BG Color"=w245, "Active Cell"=w244, "Cell BG Color"=w243) -> ()  [unwired: 2 in, 2 out]
            n132 = call <vilib>:"WPI_DashboardUpdate Command Params.vi"("Update"=w237, "NewVal"=w238, "Commands"=w236, "Param Tbl"=w235) -> ()  [unwired: 7 in, 1 out]
          }
        }
        n133 = call <vilib>:"Connextion Info.vi"() -> ("Connected"=→"NT Connection":bool)  [unwired: 10 in, 1 out]
      }
      event "Test Tree": Value Change {
        # "Show appropriate\ncontrols"
        n134 = event-data() -> ("CtlRef"=w252:refnum<vi>, "NewVal"=w250:string)  [unwired: 1 in]
        n135 = call <vilib>:"WPI_UtilitiesGetTreeIOName.vi"("NewVal"=w250, "TreeControl in"=w252) -> ("I/O Name"=w253:string)  [unwired: 9 in]
        n136 = case shown="\"Analog Out\", \"Motor\", \"PWM\"" w253 {
          selector: w253 -> [_ w260 _ w282 w291 _]
          tunnel: w250 -> [_ _ w279 w281 _ w298]
          tunnel: cluster{string[]}[] [{["640x480", "320x240", "160x120"]}, {["Auto", "Fixed indoor", "Fixed outdoor 1", "Fixed outdoor 2", "Fixed fluorescent 1", "Fixed fluorescent 2", "Hold current"]}, {["Auto", "Flicker-free 50 Hz", "Flicker-free 60 Hz", "Hold current"]}, {["None", "Prioritize frame rate", "Prioritize image quality"]}, {["Monochrome", "Color"]}] -> [_ _ _ _ _ w297]
          frame Default {
            w255 = FALSE ("Visible")
            w254 = FALSE ("Visible")
            n137 = property on="Motor" class="Clust (strict)"("Visible"=w254) -> ()  [unwired: 2 in, 2 out]
            n138 = property on="Test Ring" class="Ring (strict)"("Visible"=w254) -> ()  [unwired: 2 in, 2 out]
            n139 = property on="Rev/Fwd" class="Clust (strict)"("Visible"=w255) -> ()  [unwired: 2 in, 2 out]
            n140 = property on="On/Off" class="Bool (strict)"("Visible"=w255) -> ()  [unwired: 2 in, 2 out]
            n141 = property on="Test Slider" class="Slide (strict)"("Visible"=w255) -> ()  [unwired: 2 in, 2 out]
          }
          frame "Analog Out", "Motor", "PWM" {
            w261 = FALSE ("Visible")
            n142 = case shown="\"Analog Out\"" w260 {
              tunnel: [1.0 ("Value") -1.0 ("Value") 0.0 ("Value")] -> w259
              tunnel: [255.0 ("Value") 1.0 ("Value") 5.0 ("Value")] -> w258
              tunnel: [128.0 ("Value") 0.0 ("Value") 0.0 ("Value")] -> w257
              tunnel: [64.0 ("Value") 0.5 ("Value") 1.0 ("Value")] -> w256
              frame "PWM" {
              }
              frame "Motor", Default {
              }
              frame "Analog Out" {
              }
            }
            n143 = property on="Motor" class="Clust (strict)"("Visible"=TRUE) -> ()  [unwired: 2 in, 2 out]
            n144 = property on="Value" class="Slide (strict)"("Value"=w257, "Scale.Minimum"=w259, "Scale.Maximum"=w258, "Scale.Increment"=w256) -> ()  [unwired: 2 in, 2 out]
            n145 = property on="On/Off" class="Bool (strict)"("Visible"=w261) -> ()  [unwired: 2 in, 2 out]
            n146 = property on="Test Slider" class="Slide (strict)"("Visible"=w261) -> ()  [unwired: 2 in, 2 out]
            n147 = property on="Test Ring" class="Ring (strict)"("Visible"=w261) -> ()  [unwired: 2 in, 2 out]
            n148 = property on="Rev/Fwd" class="Clust (strict)"("Visible"=w261) -> ()  [unwired: 2 in, 2 out]
          }
          frame "Servo" {
            w277 = FALSE ("Visible")
            n149 = call <vilib>:"NT Read Number.vi"("Name"=w279) -> ("Numeric"=w278:dbl)  [unwired: 9 in, 1 out]
            n150 = property on="Test Slider" class="Slide (strict)"("Visible"=TRUE, "Scale.Maximum"=170.0 ("Scale.Range:Maximum")) -> ()  [unwired: 2 in, 2 out]
            n151 = local write "Test Slider"(w278) -> ()
            n152 = property on="Motor" class="Clust (strict)"("Visible"=w277) -> ()  [unwired: 2 in, 2 out]
            n153 = property on="Rev/Fwd" class="Clust (strict)"("Visible"=w277) -> ()  [unwired: 2 in, 2 out]
            n154 = property on="On/Off" class="Bool (strict)"("Visible"=w277) -> ()  [unwired: 2 in, 2 out]
            n155 = property on="Test Ring" class="Ring (strict)"("Visible"=w277) -> ()  [unwired: 2 in, 2 out]
          }
          frame "Relay", "Solenoid" {
            w280 = FALSE ("Visible")
            n156 = property on="Motor" class="Clust (strict)"("Visible"=w280) -> ()  [unwired: 2 in, 2 out]
            n157 = property on="Test Slider" class="Slide (strict)"("Visible"=w280) -> ()  [unwired: 2 in, 2 out]
            n158 = Search and Replace String(input string=w281, search string="/Value  **", replace string="/Direction") -> (result string=w287:string)  [unwired: 5 in, 3 out]
            n159 = property on="Test Ring" class="Ring (strict)"("Visible"=w280) -> ()  [unwired: 2 in, 2 out]
            n160 = call <vilib>:"NT Read String.vi"("Name"=w287) -> ("String"=w285:string)  [unwired: 9 in, 1 out]
            n161 = Equal?(x="Both directions", y=w285) -> (x = y?=w283:bool)
            n162 = Not(x=w283) -> (.not. x?=w284:bool)
            n163 = property on="Rev/Fwd" class="Clust (strict)"("Visible"=w283) -> ()  [unwired: 2 in, 2 out]
            n164 = property on="On/Off" class="Bool (strict)"("Visible"=w284, "Caption.Text"=w282) -> ()  [unwired: 2 in, 2 out]
          }
          frame "Compressor", "Digital Out" {
            w290 = FALSE ("Visible")
            # "Get direction and finish"
            n165 = property on="Motor" class="Clust (strict)"("Visible"=w290) -> ()  [unwired: 2 in, 2 out]
            n166 = property on="Test Slider" class="Slide (strict)"("Visible"=w290) -> ()  [unwired: 2 in, 2 out]
            n167 = property on="Test Ring" class="Ring (strict)"("Visible"=w290) -> ()  [unwired: 2 in, 2 out]
            n168 = property on="On/Off" class="Bool (strict)"("Visible"=TRUE, "Caption.Text"=w291) -> ()  [unwired: 2 in, 2 out]
            n169 = property on="Rev/Fwd" class="Clust (strict)"("Visible"=FALSE) -> ()  [unwired: 2 in, 2 out]
          }
          frame "Camera" {
            n170 = call <vilib>:"Get Last Path Segment.vi"("String in"=w298) -> ("String out"=w299:string)  [unwired: 10 in]
            n171 = property on="On/Off" class="Bool (strict)"("Visible"=FALSE) -> ()  [unwired: 2 in, 2 out]
            n172 = property on="Motor" class="Clust (strict)"("Visible"=FALSE) -> ()  [unwired: 2 in, 2 out]
            n173 = property on="Rev/Fwd" class="Clust (strict)"("Visible"=FALSE) -> ()  [unwired: 2 in, 2 out]
            n174 = case shown="\"White Balance  **\"" w299 {
              tunnel: w298 -> [w305 w314 w323 w332 w341 _ w347]
              tunnel: w297 -> [w303 w311 w320 w329 w338 _ _]
              frame "Size  **" {
                n175 = Index Array(array=w303) -> (element=w302:cluster{string[]})  [unwired: 1 in]
                n176 = call <vilib>:"NT Read String.vi"("Name"=w305) -> ("String"=w304:string)  [unwired: 9 in, 1 out]
                n177 = Unbundle(w302) -> (w300:string[])
                n178 = Match First String(2:w300, 3:w304) -> (0:w301:i32)  [unwired: 1 out]
                n179 = property on="Test Ring" class="Ring (strict)"("Value"=w301, "Strings []"=w300) -> ()  [unwired: 2 in, 2 out]
                n180 = property on="Test Ring" class="Ring (strict)"("Visible"=TRUE) -> ()  [unwired: 2 in, 2 out]
                n181 = property on="Test Slider" class="Slide (strict)"("Visible"=FALSE) -> ()  [unwired: 2 in, 2 out]
              }
              frame "White Balance  **" {
                n182 = Index Array(array=w311, index=1) -> (element=w312:cluster{string[]})
                n183 = call <vilib>:"NT Read String.vi"("Name"=w314) -> ("String"=w313:string)  [unwired: 9 in, 1 out]
                n184 = Unbundle(w312) -> (w309:string[])
                n185 = Match First String(2:w309, 3:w313) -> (0:w308:i32)  [unwired: 1 out]
                n186 = property on="Test Ring" class="Ring (strict)"("Value"=w308, "Strings []"=w309) -> ()  [unwired: 2 in, 2 out]
                n187 = property on="Test Ring" class="Ring (strict)"("Visible"=TRUE) -> ()  [unwired: 2 in, 2 out]
                n188 = property on="Test Slider" class="Slide (strict)"("Visible"=FALSE) -> ()  [unwired: 2 in, 2 out]
              }
              frame "Exposure  **" {
                n189 = Index Array(array=w320, index=2) -> (element=w321:cluster{string[]})
                n190 = call <vilib>:"NT Read String.vi"("Name"=w323) -> ("String"=w322:string)  [unwired: 9 in, 1 out]
                n191 = Unbundle(w321) -> (w317:string[])
                n192 = Match First String(2:w317, 3:w322) -> (0:w318:i32)  [unwired: 1 out]
                n193 = property on="Test Ring" class="Ring (strict)"("Value"=w318, "Strings []"=w317) -> ()  [unwired: 2 in, 2 out]
                n194 = property on="Test Ring" class="Ring (strict)"("Visible"=TRUE) -> ()  [unwired: 2 in, 2 out]
                n195 = property on="Test Slider" class="Slide (strict)"("Visible"=FALSE) -> ()  [unwired: 2 in, 2 out]
              }
              frame "Exposure Priority  **" {
                n196 = Index Array(array=w329, index=3) -> (element=w330:cluster{string[]})
                n197 = call <vilib>:"NT Read String.vi"("Name"=w332) -> ("String"=w331:string)  [unwired: 9 in, 1 out]
                n198 = Unbundle(w330) -> (w326:string[])
                n199 = Match First String(2:w326, 3:w331) -> (0:w327:i32)  [unwired: 1 out]
                n200 = property on="Test Ring" class="Ring (strict)"("Value"=w327, "Strings []"=w326) -> ()  [unwired: 2 in, 2 out]
                n201 = property on="Test Ring" class="Ring (strict)"("Visible"=TRUE) -> ()  [unwired: 2 in, 2 out]
                n202 = property on="Test Slider" class="Slide (strict)"("Visible"=FALSE) -> ()  [unwired: 2 in, 2 out]
              }
              frame "Color Enable  **" {
                n203 = Index Array(array=w338, index=4) -> (element=w339:cluster{string[]})
                n204 = call <vilib>:"NT Read String.vi"("Name"=w341) -> ("String"=w340:string)  [unwired: 9 in, 1 out]
                n205 = Unbundle(w339) -> (w335:string[])
                n206 = Match First String(2:w335, 3:w340) -> (0:w336:i32)  [unwired: 1 out]
                n207 = property on="Test Ring" class="Ring (strict)"("Value"=w336, "Strings []"=w335) -> ()  [unwired: 2 in, 2 out]
                n208 = property on="Test Ring" class="Ring (strict)"("Visible"=TRUE) -> ()  [unwired: 2 in, 2 out]
                n209 = property on="Test Slider" class="Slide (strict)"("Visible"=FALSE) -> ()  [unwired: 2 in, 2 out]
              }
              frame Default {
                n210 = property on="Test Ring" class="Ring (strict)"("Visible"=FALSE) -> ()  [unwired: 2 in, 2 out]
                n211 = property on="Test Slider" class="Slide (strict)"("Visible"=FALSE) -> ()  [unwired: 2 in, 2 out]
              }
              frame "Brightness  **", "Color Level  **", "Compression  **", "FPS  **", "Sharpness  **" {
                n212 = call <vilib>:"NT Read Number.vi"("Name"=w347) -> ("Numeric"=w346:dbl)  [unwired: 9 in, 1 out]
                n213 = local write "Test Slider"(w346) -> ()
                n214 = property on="Test Slider" class="Slide (strict)"("Visible"=TRUE, "Scale.Maximum"=100.0 ("Scale.Range:Maximum")) -> ()  [unwired: 2 in, 2 out]
                n215 = property on="Test Ring" class="Ring (strict)"("Visible"=FALSE) -> ()  [unwired: 2 in, 2 out]
              }
            }
          }
        }
        n216 = property on="Progress" class="Clust (strict)"("Visible"=FALSE) -> ()  [unwired: 2 in, 2 out]
      }
      event "Test Name": Mouse Enter {
        # "Populate the ring with the list of tests"
        n217 = event-data() -> ()  [unwired: 1 in, 1 out]
        n218 = call <vilib>:"NT Read String Array.vi"("Name"="TestMode/TestList") -> ("String Array"=w355:string[])  [unwired: 9 in, 1 out]
        n219 = Build Array (concatenate)("Select the test to run...", w355) -> (w354:string[])
        n220 = property on="Test Name" class="Ring (strict)"("Strings []"=w354) -> ()  [unwired: 2 in, 2 out]
      }
      event "Test Name": Value Change {
        w357 = FALSE ("Visible")
        # "Tell the robot the test name to run"
        n221 = event-data() -> ("NewVal"=w361:u16)  [unwired: 1 in]
        n222 = property on="Test Name" class="Ring (strict)"() -> ("Strings []"=w362:string[])  [unwired: 2 in, 2 out]
        n223 = local write "Progress"(T6 {"Test Progress"=0, "Test Progress Text"=""} ("Progress")) -> ()
        n224 = Index Array(array=w362, index=w361) -> (element=w360:string)
        n225 = call <vilib>:"NT Write String.vi"("String"=w360, "Name"="TestMode/TestName") -> ()  [unwired: 9 in, 1 out]
        n226 = property on="Progress" class="Clust (strict)"("Visible"=TRUE) -> ()  [unwired: 2 in, 2 out]
        n227 = property on="Motor" class="Clust (strict)"("Visible"=w357) -> ()  [unwired: 2 in, 2 out]
        n228 = property on="Test Slider" class="Slide (strict)"("Visible"=w357) -> ()  [unwired: 2 in, 2 out]
        n229 = property on="On/Off" class="Bool (strict)"("Visible"=w357) -> ()  [unwired: 2 in, 2 out]
        n230 = property on="Rev/Fwd" class="Clust (strict)"("Visible"=w357) -> ()  [unwired: 2 in, 2 out]
        n231 = property on="Test Ring" class="Ring (strict)"("Visible"=w357) -> ()  [unwired: 2 in, 2 out]
      }
      event "Select Auto": Mouse Enter {
        # "Populate the combo box with the list of autonomous options"
        n232 = event-data() -> ()  [unwired: 1 in, 1 out]
        n233 = call <vilib>:"NT Read String Array.vi"("Name"="Auto List") -> ("String Array"=w364:string[])  [unwired: 9 in, 1 out]
        n234 = property on="Select Auto" class="CmbBox"("Strings[]"=w364) -> ()  [unwired: 2 in, 2 out]
      }
      event "Select Auto": Value Change {
        # "User modified the Auto Selection. Write to NT variable so robot knows."
        n235 = event-data() -> ("NewVal"=w367:string)  [unwired: 1 in]
        n236 = call <vilib>:"NT Write String.vi"("String"=w367, "Name"="Auto Selector") -> ()  [unwired: 9 in, 1 out]
      }
      event "Command Selection": Value Change {
        # "Get the params and show in table"
        n237 = event-data() -> ("NewVal"=w373:i32)  [unwired: 1 in]
        n238 = property on="Command Selection" class="MCListbox (strict)"() -> ("ItemNames"=w371:string[][])  [unwired: 2 in, 2 out]
        n239 = call <vilib>:"WPI_DashboardUpdate Command Params.vi"("NewVal"=w373, "Commands"=w371, "Param Tbl"=w372) -> ()  [unwired: 8 in, 1 out]
      }
      event "Execute Command": Value Change {
        # "Started one, Unique ID holds\nresponse"
        n240 = event-data() -> ()  [unwired: 1 in, 1 out]
        n241 = property on="Command Selection" class="MCListbox (strict)"() -> ("ItemNames"=w384:string[][])  [unwired: 2 in, 2 out]
        n242 = Index Array(array=w384, index (row)="Command Selection", index (col)=0) -> (element=w382:string)
        n243 = call <vilib>:"Invoke Commands.vi"("Command Params"="Command Params", "Function Name"=w382) -> ("Params"=w378:u8, "Started"=w377:bool)  [unwired: 7 in, 1 out]
        n244 = Array Subset(array="Command Params", length (row)=w378) -> (w379:string[][])  [unwired: 3 in]
        n245 = Select(t="Executing" ("Cmd Status"), s=w377, f="" ("Cmd Status")) -> (s? t:f=→"Cmd Status":string)
      }
      event "Command Selection": Double Click {
        n246 = event-data() -> ("Row"=w392:i32)  [unwired: 1 in]
        n247 = property on="Command Selection" class="MCListbox (strict)"() -> ("ItemNames"=w395:string[][])  [unwired: 2 in, 2 out]
        n248 = local read "Command Params"() -> (w391:string[][])
        n249 = Index Array(array=w395, index (row)=w392, index (col)=0) -> (element=w393:string)
        n250 = call <vilib>:"Invoke Commands.vi"("Command Params"=w391, "Function Name"=w393) -> ("Params"=w390:u8, "Started"=w385:bool)  [unwired: 7 in, 1 out]
        n251 = Array Subset(array=w391, length (row)=w390) -> (w389:string[][])  [unwired: 3 in]
        n252 = Select(t="Executing" ("Cmd Status"), s=w385, f="" ("Cmd Status")) -> (s? t:f=w386:string)
        n253 = local write "Cmd Status"(w386) -> ()
      }
      event "CheckList": Double Click {
        # "Shift clears all"
        # "Update symbols on the listbox"
        n254 = event-data() -> ("PlatMods.Shift"=w397:bool, "Row"=w399:i32)  [unwired: 1 in]
        n255 = case shown="True" w397 {
          tunnel: w399 -> [w403 _]
          tunnel: 1 -> [w402 _]
          frame False {
            n256 = property on="CheckList" class="LstBox (strict)"() -> ("Item Symbols"=w401:i32[])  [unwired: 2 in, 2 out]
            n257 = Replace Array Subset(array=w401, new element=w402, index=w403) -> (w400:i32[])
            n258 = property on="CheckList" class="LstBox (strict)"("Item Symbols"=w400) -> ()  [unwired: 2 in, 2 out]
          }
          frame True {
            w404 = 0 ("Top Row")
            n259 = property on="CheckList" class="LstBox (strict)"() -> ("Number of Rows"=w406:u32)  [unwired: 2 in, 2 out]
            n260 = Initialize Array(0, w406) -> (w405:i32[])
            n261 = property on="CheckList" class="LstBox (strict)"("Top Row"=w404, "Value"=w404, "Item Symbols"=w405) -> ()  [unwired: 2 in, 2 out]
          }
        }
      }
      event "CheckList": Key Down {
        # "Update symbols on the listbox\nLeft and right keys check and uncheck"
        n262 = event-data() -> ("VKey"=w410:T23)  [unwired: 1 in]
        n263 = case shown="\"Left\", \"Right\"" w410 {
          selector: w410 -> [w415 _]
          tunnel: eventvkey."Left" ("VKey") -> [w413 _]
          frame "Left", "Right" {
            n264 = Equal?(x=w413, y=w415) -> (x = y?=w414:bool)
            n265 = Select(t=0, s=w414, f=1) -> (s? t:f=w416:i32)
            n266 = property on="CheckList" class="LstBox (strict)"() -> ("Item Symbols"=w419:i32[])  [unwired: 2 in, 2 out]
            n267 = Replace Array Subset(array=w419, new element=w416, index="CheckList") -> (w418:i32[])
            n268 = property on="CheckList" class="LstBox (strict)"("Item Symbols"=w418) -> ()  [unwired: 2 in, 2 out]
          }
          frame Default {
          }
        }
      }
      event "Motor.Enable": Value Change {
        # "When the test mode otor enable helper is set, update that\ntree row item's value"
        n269 = event-data() -> ("NewVal"=w425:bool)  [unwired: 1 in]
        n270 = Unbundle("Motor") -> ("Value"=w424:dbl)  [unwired: 1 out]
        n271 = Select(t=w424, s=w425, f=0.0) -> (s? t:f=w422:dbl)
        n272 = call <vilib>:"NT Write Number.vi"("Numeric"=w422, "Name"=w421) -> ()  [unwired: 9 in, 1 out]
      }
      event "Test Slider": Value Change {
        # "When the test mode slider helper is set, update that\ntree row item's value"
        n273 = event-data() -> ("NewVal"=w428:dbl)  [unwired: 1 in]
        n274 = call <vilib>:"NT Write Number.vi"("Numeric"=w428, "Name"=w429) -> ()  [unwired: 9 in, 1 out]
      }
      event "On/Off": Value Change {
        # "When the test mode on/off helper value is set, update that\ntree row item's value"
        n275 = event-data() -> ("NewVal"=w433:bool)  [unwired: 1 in]
        n276 = Boolean To (0,1)(Boolean=w433) -> (0, 1=w432:i16)
        n277 = call <vilib>:"NT Write Number.vi"("Numeric"=w432, "Name"=w431) -> ()  [unwired: 9 in, 1 out]
      }
      event "Rev/Fwd": Value Change {
        # "When the test mode helper value for relays is set, update that\ntree row item's value"
        n278 = event-data() -> ("NewVal.Forward"=w441:bool, "NewVal.Reverse"=w440:bool)  [unwired: 1 in]
        n279 = Boolean To (0,1)(Boolean=w441) -> (0, 1=w437:i16)
        n280 = Boolean To (0,1)(Boolean=w440) -> (0, 1=w439:i16)
        n281 = Negate(x=w439) -> (-x=w438:i16)
        n282 = Add(x=w437, y=w438) -> (x+y=w436:i16)
        n283 = call <vilib>:"NT Write Number.vi"("Numeric"=w436, "Name"=w435) -> ()  [unwired: 9 in, 1 out]
      }
      event "Test Ring": Value Change {
        # "When a test mode helper value is selected from the ring,\nset the tree item's variable to the string value"
        n284 = event-data() -> ("NewVal"=w445:u16)  [unwired: 1 in]
        n285 = property on="Test Ring" class="Ring (strict)"() -> ("Strings []"=w446:string[])  [unwired: 2 in, 2 out]
        n286 = Index Array(array=w446, index=w445) -> (element=w444:string)
        n287 = call <vilib>:"NT Write String.vi"("String"=w444, "Name"=w443) -> ()  [unwired: 9 in, 1 out]
      }
      event "Rec Mode": Value Change {
        # "Update globals for recording mode and path to read log from.\nClear when logging and let NetworkTables set path for vision to\nuse."
        n288 = event-data() -> ("NewVal"=w457:enum32{"Stop", "Record", "Playback"})  [unwired: 1 in]
        n289 = global write "WPI_DashboardLogging Global.vi" "Logging Filename"(path "") -> ()
        n290 = global write "WPI_DashboardLogging Global.vi" "Recording"(w457) -> ()
        n291 = case shown="\"Playback\"" w457 {
          tunnel: w456 -> [_ w459 w468]
          tunnel: [_ _ w467] -> w454
          tunnel: [_ _ w466] -> _
          tunnel: w452 -> [_ _ w464]
          tunnel: cluster{i32, i32} {-250, 170} -> [_ _ w463]
          tunnel: [_ _ T24 {"Image Size"=TRUE, "Image Type"=TRUE, "Pixel Value"=TRUE, "ROI Information"=TRUE, "Zoom Factor"=FALSE} ("Image Information Shown:All Elements")] -> w447
          tunnel: [_ _ TRUE ("Zoom Factor")] -> w448
          tunnel: w450 -> [_ _ w460]
          frame Default {
          }
          frame "Stop", "Record" {
            # "Place Window too"
            n292 = invoke class="VI" method="FP.Close"(reference=w459) -> (reference out=w458:refnum<vi>)  [unwired: 2 in, 2 out]
            n293 = invoke class="VI" method="Abort VI"(reference=w458) -> ()  [unwired: 2 in, 3 out]
          }
          frame "Playback" {
            n294 = call "Open Playback Panel.vi"("Offset"=w463, "DB VI Ref"=w464, "Playback in"=w468) -> ("Playback out"=w465:refnum<vi>)  [unwired: 8 in]
            n295 = register-events(w465, w460) -> (reference out=w467:refnum<event-registration>, error out=w466:errorcluster)  [unwired: 2 in]
          }
        }
        n296 = property on="Camera Image Right" class="ImageControl"("Image Information Shown"=w447, "Image Information Visible"=w448) -> ()  [unwired: 2 in, 2 out]
        n297 = property on="Camera Image" class="ImageControl"("Image Information Shown"=w447, "Image Information Visible"=w448) -> ()  [unwired: 2 in, 2 out]
        n298 = call <vilib>:"WPI_DashboardNT Log FieldName Cache.vi"("Operation"=enum16{"Lookup/Add", "Index", "Clear"}."Clear") -> ()  [unwired: 8 in, 3 out]
      }
      event Panel Close {
        w470 = enum32{"Stop", "Record", "Playback"}."Stop" ("Rec Mode")
        # "Playback window has been closed, abort"
        n299 = event-data() -> ()  [unwired: 1 in, 4 out]
        n300 = local write "Rec Mode"(w470) -> ()
        n301 = global write "WPI_DashboardLogging Global.vi" "Recording"(w470) -> ()
      }
      event Panel Close {
        # "Abort playback window and ourself"
        n302 = event-data() -> ()  [unwired: 1 in, 4 out]
        n303 = invoke class="VI" method="FP.Close"(reference=w474) -> (reference out=w473:refnum<vi>)  [unwired: 2 in, 2 out]
        n304 = invoke class="VI" method="Abort VI"(reference=w473) -> (error out=w472:errorcluster)  [unwired: 2 in, 2 out]
        n305 = invoke class="VI" method="Abort VI"(error in=w472) -> ()  [unwired: 2 in, 3 out]
      }
      event User Event {
        n306 = event-data() -> ("IDs"=w481:cluster{"RPC field ID":u16, "Unique ID":u16}, "String"=w480:string)  [unwired: 1 in]
        n307 = Bundle("IDs"=w481, "String"=w480) -> (w479:T10)  [unwired: 1 in]
        n308 = call <vilib>:"Retrieve RPC Response.vi"("RPC Response"=w479) -> ("Output"=w477:string[][])  [unwired: 10 in]
        n309 = Build Array (concatenate)(w475, w477) -> (w476:string[][])
        n310 = local write "Command Params"(w476) -> ()
        n311 = local write "Cmd Status"("" ("Cmd Status")) -> ()
      }
      event "Tree": Double Click {
        n312 = event-data() -> ("PlatMods"=w487:T27, "Tag"=w484:string)  [unwired: 1 in]
        n313 = Unbundle(w487) -> ("Shift"=w486:bool)  [unwired: 4 out]
        n314 = String Subset(string=w484, length (rest)=1 ("length (rest)")) -> (substring=w483:string)  [unwired: 1 in]
        n315 = Not(x=w486) -> (.not. x?=w485:bool)
        n316 = case shown="\"/\"" w483 {
          tunnel: w484 -> [_ w490]
          tunnel: w485 -> [_ w489]
          frame Default {
          }
          frame "/" {
            n317 = call <vilib>:"NT Update Persistence.vi"("Persistence"=w489, "Name"=w490) -> ()  [unwired: 9 in, 1 out]
          }
        }
      }
    }
  }
  n318 = while {
    tunnel: w65 -> [w492]
    i -> [w495]
    stop <- FALSE stop-if-true
    n319 = Wait (ms)(milliseconds to wait=u32 100) -> ()  [unwired: 1 out]
    n320 = case shown="\"Playback\"" "Rec Mode" {
      tunnel: w495 -> [_ _ w510]
      tunnel: [u32 2829099 ("Base Color") u32 11141120 ("Target Color") w499] -> w491
      frame "Stop", Default {
        # "Reset the color, extra updates don't cost much"
      }
      frame "Record" {
      }
      frame "Playback" {
        # "Playback"
        n321 = Quotient & Remainder(x=w510, y=u32 50 ("milliseconds to wait")) -> (x-y*floor(x/y)=w506:u32)  [unwired: 1 out]
        n322 = Divide(x=w506, y=u32 50 ("milliseconds to wait")) -> (x/y=w503:dbl)
        n323 = Multiply(x=6.283185307179586, y=w503) -> (x*y=w508:dbl)
        n324 = Sine(x=w508) -> (sin(x)=w507:dbl)
        n325 = Absolute Value(x=w507) -> (abs(x)=w500:dbl)
        n326 = call "Interpolate RGB Color.vi"("Proportion"=w500, "Target Color"=u32 30976, "Base Color"=u32 2829099) -> ("Result Color"=w499:u32)  [unwired: 8 in]
      }
    }
    n327 = property class="Pane"(reference=w492, "PaneColor"=w491) -> ()  [unwired: 1 in, 2 out]
  }
  n328 = local write "Dashboard Tab"(T2."Operation" ("Dashboard Tab")) -> ()
  n329 = property on="On/Off" class="Bool (strict)"("Visible"=w36) -> ()  [unwired: 2 in, 2 out]
  n330 = property on="Motor" class="Clust (strict)"("Visible"=w36) -> ()  [unwired: 2 in, 2 out]
  n331 = property on="Progress" class="Clust (strict)"("Visible"=w36) -> ()  [unwired: 2 in, 2 out]
  n332 = property on="Test Ring" class="Ring (strict)"("Visible"=w36) -> ()  [unwired: 2 in, 2 out]
  n333 = property on="Rev/Fwd" class="Clust (strict)"("Visible"=w36) -> ()  [unwired: 2 in, 2 out]
  n334 = while {
    tunnel: u16 1741 ("timeout ms (25000)") -> [w512]
    stop <- FALSE stop-if-true
    n335 = TCP Create Listener(10:w512) -> (0:w511:errorcluster, 3:w513:refnum<k5>)  [unwired: 4 in, 1 out]
    n336 = case shown="No Error" w511 {
      selector: w511 -> [w515 _]
      tunnel: w513 -> [w516 _]
      frame No Error {
        n337 = while {
          tunnel: w516 -> [w519]
          tunnel: w515 -> [w518]
          stop <- FALSE stop-if-true
          n338 = TCP Wait On Listener(8:w518, 11:w519) -> (0:w520:errorcluster, 4:w521:refnum<k5>)  [unwired: 2 in, 3 out]
          n339 = local write "TCP"(w521) -> ()
          n340 = case shown="No Error" w520 {
            frame No Error {
            }
            frame Error {
              n341 = Wait (ms)(milliseconds to wait=u32 1000) -> ()  [unwired: 1 out]
            }
          }
        }
      }
      frame Error {
        n342 = Wait (ms)(milliseconds to wait=u32 1000) -> ()  [unwired: 1 out]
      }
    }
  }
  n343 = local write "Command Selection"(u16 0 ("milliseconds to wait")) -> ()
  n344 = local write "Command Params"(string[][] [] ("Command Params")) -> ()
  n345 = global write "WPI_DashboardLogging Global.vi" "Recording"(w59) -> ()
  n346 = local write "Rec Mode"(w59) -> ()
  n347 = call <vilib>:"NT Write String.vi"("String"="Select Auto", "Name"="Auto Selector") -> ()  [unwired: 9 in, 1 out]
  n348 = while {
    stop <- FALSE stop-if-true
    # "Limelight Variables"
    n349 = Wait (ms)(milliseconds to wait=u32 50) -> ()  [unwired: 1 out]
    n350 = call-poly <vilib>:"NT Read Value.vi"("Default Value"=0.0, "Name"="Top RPM") -> ("Numeric"=w534:dbl)  [unwired: 8 in, 1 out]
    n351 = call-poly <vilib>:"NT Read Value.vi"("Name"="/limelight/ty") -> ("Numeric"=→"Offset Y":dbl)  [unwired: 9 in, 1 out]
    n352 = call-poly <vilib>:"NT Read Value.vi"("Name"="/limelight/tx") -> ("Numeric"=→"Offset X":dbl)  [unwired: 9 in, 1 out]
    n353 = call-poly <vilib>:"NT Read Value.vi"("Name"="/limelight/ts") -> ("Numeric"=→"Skew":dbl)  [unwired: 9 in, 1 out]
    n354 = call-poly <vilib>:"NT Read Value.vi"("Name"="/limelight/ta") -> ("Numeric"=→"Area":dbl)  [unwired: 9 in, 1 out]
    n355 = call-poly <vilib>:"NT Read Value.vi"("Default Value"=0.0, "Name"="Bottom RPM") -> ("Numeric"=w532:dbl)  [unwired: 8 in, 1 out]
    n356 = Round To Nearest(number=w534) -> (nearest integer value=→"Top RPM":dbl)
    n357 = Round To Nearest(number=w532) -> (nearest integer value=→"Bottom RPM":dbl)
  }
